vi "image2data_4d.vi"(10 "image_1d":sgl[](array[numeric]), 11 "Data":T1 {"slice orientation" items=["transverse unflipped", "coronal unflipped", "sagittal unflipped", "transverse flipped", "coronal flipped", "sagittal flipped"]}) -> (2 "image_4d":sgl[][][][](array[numeric]), 3 "Data":T1 {"slice orientation" items=["transverse unflipped", "coronal unflipped", "sagittal unflipped", "transverse flipped", "coronal flipped", "sagittal flipped"]})   [LabVIEW 2014]
uses:
  control/head_data.ctl
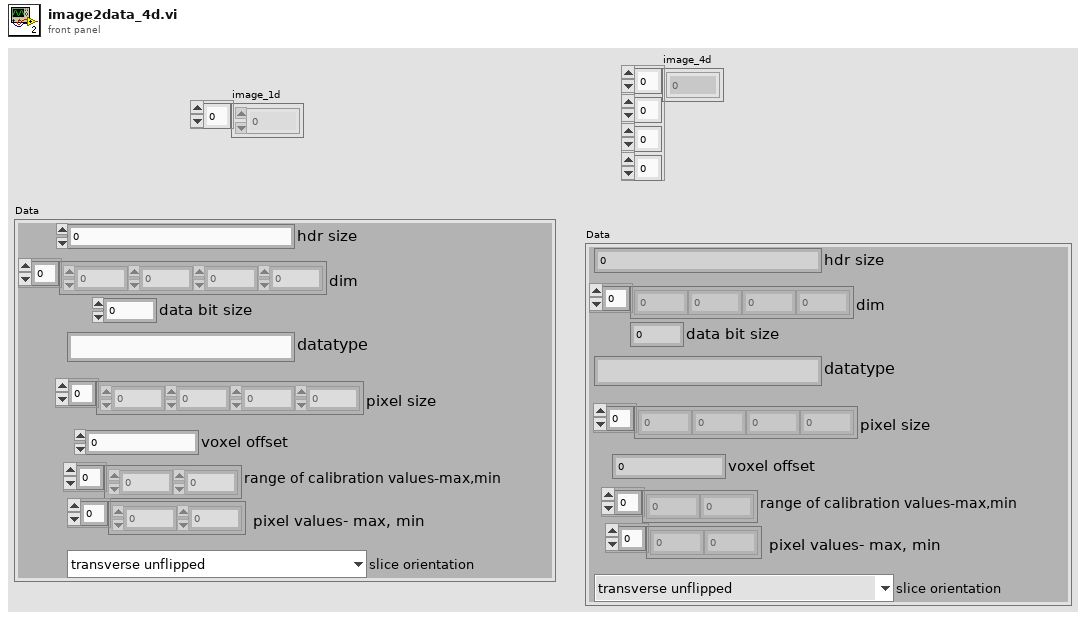
[diagram p1: front panel]
types:
  T1 = typedef "head_data.ctl" = cluster{"hdr size":i32, "dim":i32[], "data bit size":i32, "datatype":string, "pixel size ":sgl[], "voxel offset":sgl, "range of calibration values-max,min":sgl[], " pixel values- max, min":sgl[], "slice orientation":u16}
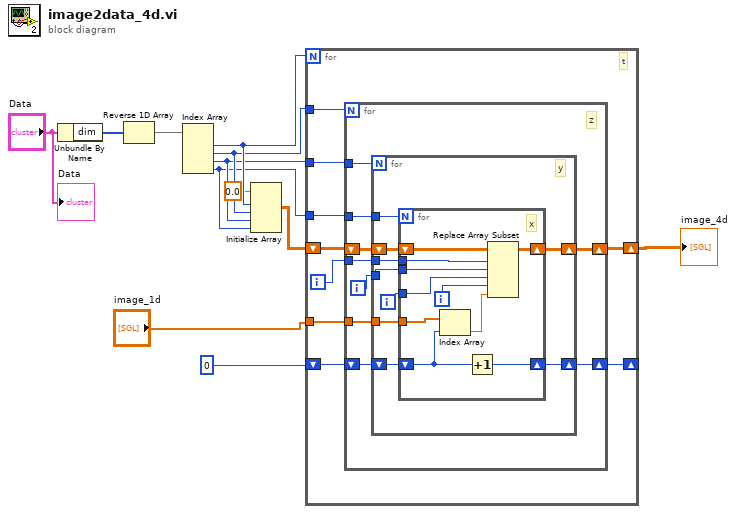
[diagram p0: block diagram]
diagram:
  n1 = Unbundle By Name("Data") -> ("dim"=w2:i32[])
  n2 = Reverse 1D Array(array=w2) -> (reversed array=w1:i32[])
  n3 = Index Array(array=w1) -> (element #1=w9:i32, element #2=w8:i32, element #3=w7:i32, element #4=w6:i32)  [unwired: 4 in]
  n4 = Initialize Array(sgl 0.0 ("element"), w9, w8, w7, w6) -> (w4:sgl[][][][])
  n5 = for {
    N: w9 -> [_]
    tunnel: "image_1d" -> [w21]
    tunnel: w6 -> [w19]
    tunnel: w7 -> [w18]
    tunnel: w8 -> [w17]
    shift-right: [w16] -> _
    shift-left: 0 -> [w20]
    shift-right: [w14] -> w3
    shift-left: w4 -> [w15]
    i -> [w13]
    # "t"
    n6 = for {
      N: w17 -> [_]
      tunnel: w21 -> [w30]
      shift-right: [w29] -> w16
      shift-left: w20 -> [w28]
      tunnel: w19 -> [w27]
      tunnel: w18 -> [w26]
      shift-right: [w24] -> w14
      shift-left: w15 -> [w25]
      tunnel: w13 -> [w22]
      i -> [w23]
      # "z"
      n7 = for {
        N: w26 -> [_]
        tunnel: w30 -> [w39]
        shift-right: [w38] -> w29
        shift-left: w28 -> [w37]
        tunnel: w27 -> [w36]
        shift-right: [w34] -> w24
        shift-left: w25 -> [w35]
        tunnel: w23 -> [w32]
        tunnel: w22 -> [w31]
        i -> [w33]
        # "y"
        n8 = for {
          N: w36 -> [_]
          tunnel: w39 -> [w49]
          shift-right: [w48] -> w38
          shift-left: w37 -> [w47]
          shift-right: [w45] -> w34
          shift-left: w35 -> [w46]
          tunnel: w33 -> [w42]
          tunnel: w32 -> [w41]
          tunnel: w31 -> [w40]
          i -> [w43]
          # "x"
          n9 = Index Array(array=w49, index=w47) -> (element=w44:sgl)
          n10 = Increment(x=w47) -> (x+1=w48:i32)
          n11 = Replace Array Subset(array=w46, new element=w44, index (dim 0)=w40, index (dim 1)=w41, index (dim 2)=w42, index (dim 3)=w43) -> (w45:sgl[][][][])
        }
      }
    }
  }
  "image_4d" <- w3
  "Data" <- "Data"
